vi "main.vi"() -> ()   [LabVIEW 2016, in "Server Controller.lvlib" / "Server Controller.lvclass"]
uses:
  Server Controller.lvclass
  \\Mac\Home/Documents/MAL-Framework/user.lib/Common Components/Controller/Controller.lvclass
  C:/Program Files (x86)/National Instruments/LabVIEW 2016/vi.lib/ActorFramework/Actor/Actor.lvclass
  UI/Server UI.lvclass
  \\Mac\Home/Documents/MAL-Framework/user.lib/Common Components/User Interface/UI.lvclass
  Server Config.lvclass
  C:/Program Files (x86)/National Instruments/LabVIEW 2016/user.lib/Configuration Dialog Actor/Configuration.lvclass
  MAL-Framework/user.lib/Common Components/Controller/Controller.lvclass
  <vilib>/ActorFramework/Actor/Actor.lvclass
panel:
  in  "Cancel Button":bool
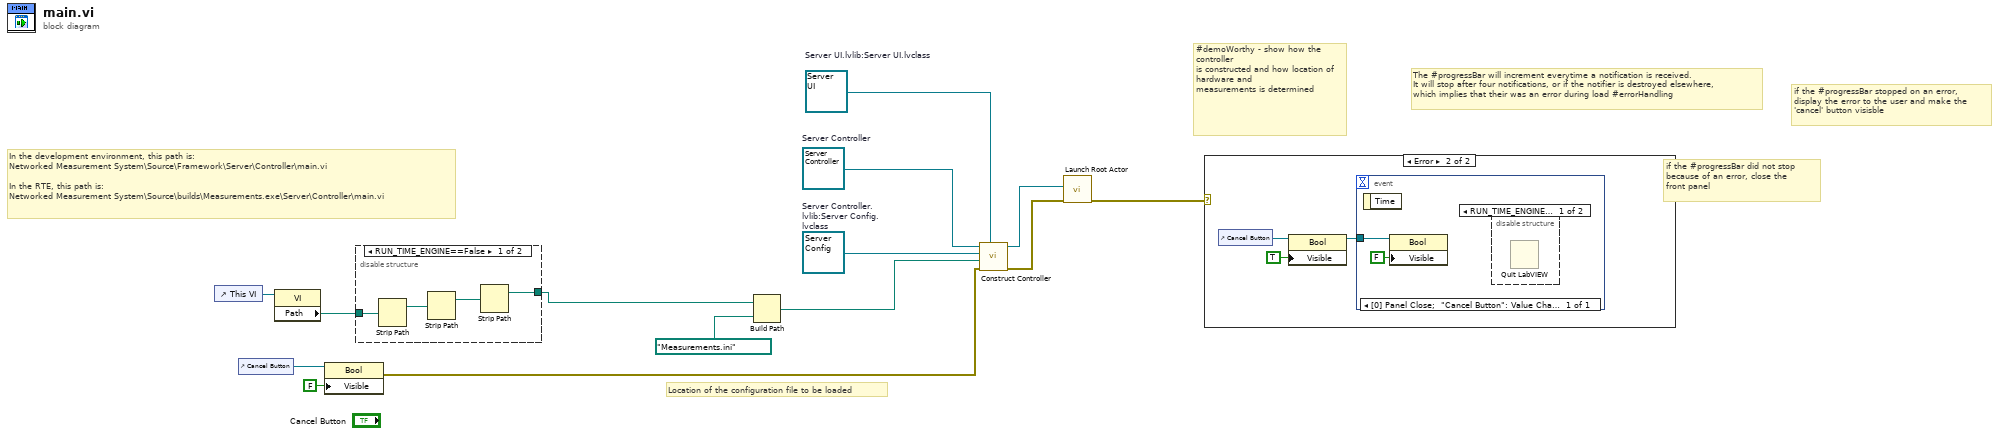
[diagram p0: block diagram]
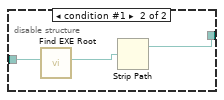
[diagram p2: hidden frame]
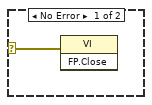
[diagram p3: hidden frame]
diagram:
  w6 = refnum<class "Server Config.lvclass"> refnum  # Server Controller.lvlib:Server Config.lvclass
  w5 = refnum<class "Server UI.lvclass"> refnum  # Server UI.lvlib:Server UI.lvclass
  w4 = refnum<class "Server Controller.lvclass"> refnum  # Server Controller
  # "Location of the configuration file to be loaded"
  # "In the development environment, this path is: \nNetworked Measurement System\\Source\\Framework\\Server\\Controller\\main.vi\n\nIn the RTE, this path is:\nNetworked Measurement System\\Source\\builds\\Measurements.exe\\Server\\Controller\\main.vi"
  # "#demoWorthy - show how the controller \nis constructed and how location of hardware and \nmeasurements is determined"
  # "if the #progressBar stopped on an error,\ndisplay the error to the user and make the\n'cancel' button visisble"
  # "if the #progressBar did not stop\nbecause of an error, close the \nfront panel"
  # "The #progressBar will increment everytime a notification is received.\nIt will stop after four notifications, or if the notifier is destroyed elsewhere,\nwhich implies that their was an error during load #errorHandling"
  n1 = control-ref of="This VI"() -> (w12:refnum<vi>)
  n2 = control-ref of="Cancel Button"() -> (w14:refnum<vi>)
  n3 = property class="VI"(reference=w12) -> ("Path"=w11:path)  [unwired: 1 in, 2 out]
  n4 = property class="Bool"(reference=w14, "Visible"=FALSE) -> (error out=w2:errorcluster)  [unwired: 1 in, 1 out]
  n5 = disable-structure shown="RUN_TIME_ENGINE==False" {
    disable-tunnel: w11 -> [w17 w21]
    disable-tunnel: [w15 w19] -> w8
    frame condition #0 (active) {
      n6 = Strip Path(path=w17) -> (stripped path=w18:path)  [unwired: 1 out]
      n7 = Strip Path(path=w18) -> (stripped path=w16:path)  [unwired: 1 out]
      n8 = Strip Path(path=w16) -> (stripped path=w15:path)  [unwired: 1 out]
    }
    frame condition #1 {
      n9 = call "Find EXE Root.vi"("Path"=w21) -> ("Location of EXE"=w20:path)  [unwired: 10 in]
      n10 = Strip Path(path=w20) -> (stripped path=w19:path)  [unwired: 1 out]
    }
  }
  n11 = Build Path(base path=w8, name or relative path=path "Measurements.ini" ("VI Path")) -> (appended path=w7:path)
  n12 = call "Construct Controller.vi"("UI.lvclass"=w5, "error in (no error)"=w2, "Root Path"=w7, "Configuration.lvlib:Configuration.lvclass"=w6, "Controller Actor.lvlib:Controller.lvclass"=w4) -> ("error out"=w1:errorcluster, "Controller Actor.lvlib:Controller.lvclass 2"=w3:refnum<class "Server Controller.lvclass">)  [unwired: 4 in, 1 out]
  n13 = call <vilib>:"Launch Root Actor.vi"("error in (no error)"=w1, "Actor"=w3) -> ("error out"=w10:errorcluster)  [unwired: 8 in, 1 out]
  n14 = case shown="Error" w10 {
    selector: w10 -> [w22 _]
    frame No Error {
      n15 = invoke class="VI" method="FP.Close"(error in=w22) -> ()  [unwired: 2 in, 3 out]
    }
    frame Error {
      n16 = control-ref of="Cancel Button"() -> (w24:refnum<vi>)
      n17 = property class="Bool"(reference=w24, "Visible"=TRUE) -> (reference out=w23:refnum<vi>)  [unwired: 1 in, 1 out]
      n18 = event shown="[0] Panel Close;  \"Cancel Button\": Value Change" {
        selector: _ -> [_]
        dyn-events: _ -> [_]
        timeout: _ -> [_]
        tunnel: w23 -> [w27]
        event Panel Close; "Cancel Button": Value Change {
          n19 = event-data() -> ()  [unwired: 1 in, 1 out]
          n20 = property class="Bool"(reference=w27, "Visible"=FALSE) -> ()  [unwired: 1 in, 2 out]
          n21 = disable-structure shown="RUN_TIME_ENGINE==True" {
            frame condition #0 {
              n22 = Quit LabVIEW() -> ()  [unwired: 1 in]
            }
            frame condition #1 (active) {
            }
          }
        }
      }
    }
  }
